vi "Agilent34410A Set AutoRange.vi"(8 "error in (no error)":errorcluster, 9 "AutoRange":bool, 10 "DMM Function":T1, 11 "VISA Rsrc":refnum<visa-resource-name>="SR530") -> (0 "error out":errorcluster, 3 "VISA Rsrc Out":refnum<visa-resource-name>="GPIB0::12::INSTR", 4 "ChaineCom":string caption="Chaîne de commande")   [LabVIEW 2019]
uses:
  <userlib>/Agilent34410A/Agilent34410A DMM_Func.ctl
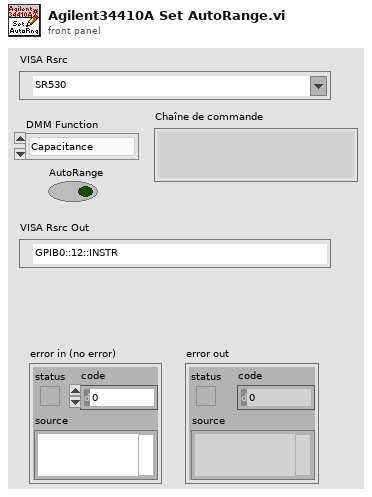
[diagram p1: front panel]
types:
  T1 = typedef "Agilent34410A DMM_Func.ctl" = enum16{"Capacitance", "Continuity", "Current AC", "Current", "Diode", "Frequency", "4W Resistance", "Period", "Resistance", "Temperature", "Voltage AC", "Voltage"}
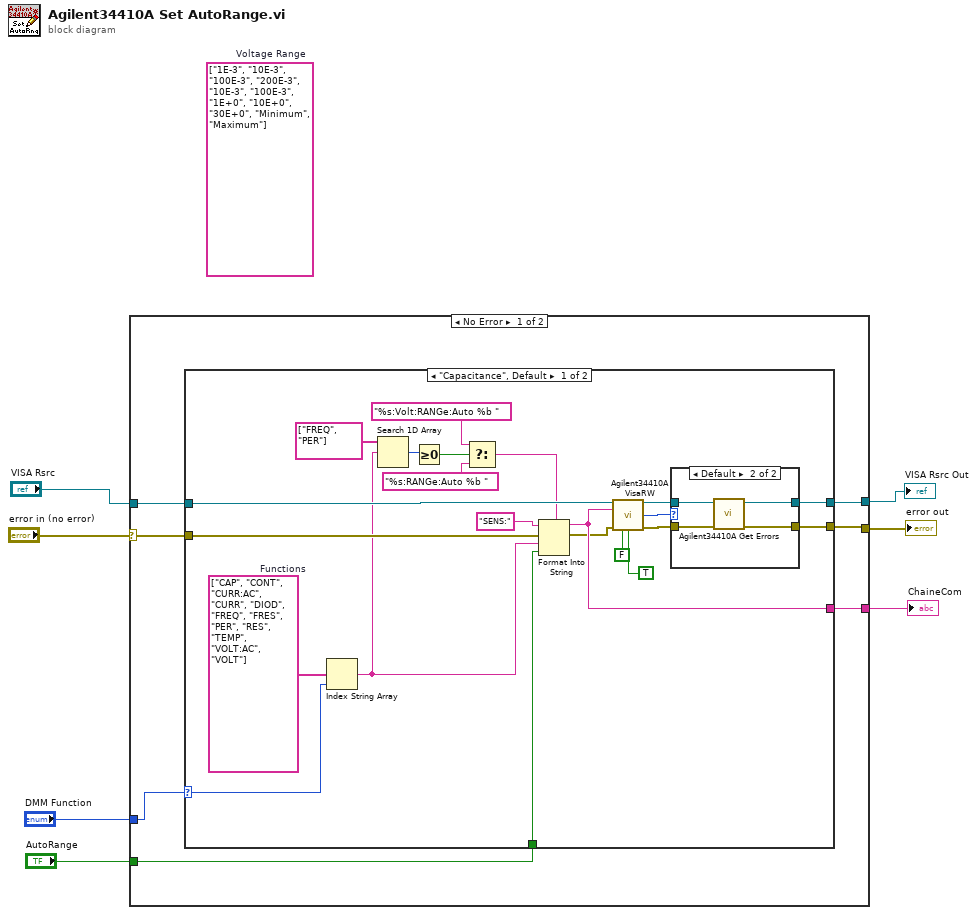
[diagram p0: block diagram]
diagram:
  (unwired) string[] ["1E-3", "10E-3", "100E-3", "200E-3", "10E-3", "100E-3", "1E+0", "10E+0", "30E+0", "Minimum", "Maximum"]  # Voltage Range
  n1 = case shown="No Error" "error in (no error)" {
    selector: "error in (no error)" -> [w12 w45]
    tunnel: "VISA Rsrc" -> [w14 w46]
    tunnel: [w11 w45] -> w5
    tunnel: [w10 w46] -> w4
    tunnel: [w13 _] -> w3
    tunnel: "DMM Function" -> [w8 _]
    tunnel: "AutoRange" -> [w9 _]
    frame No Error {
      n2 = case shown="\"Capacitance\", Default" w8 {
        selector: w8 -> [w16 _]
        tunnel: w14 -> [w36 w43]
        tunnel: [w32 _] -> w13
        tunnel: w12 -> [w31 w44]
        tunnel: [w26 w44] -> w11
        tunnel: [w25 w43] -> w10
        tunnel: w9 -> [w17 _]
        frame "Capacitance", Default {
          w35 = string[] ["CAP", "CONT", "CURR:AC", "CURR", "DIOD", "FREQ", "FRES", "PER", "RES", "TEMP", "VOLT:AC", "VOLT"]  # Functions
          n3 = Index String Array(1:w16, 2:w35) -> (0:w19:string)  [unwired: 1 in]
          n4 = Search 1D Array(1D array=string[] ["FREQ", "PER"], element=w19) -> (index of element=w23:i32)  [unwired: 1 in]
          n5 = Greater Or Equal To 0?(x=w23) -> (x >= 0?=w20:bool)
          n6 = Select(t="%s:Volt:RANGe:Auto %b " ("string (\"\")"), s=w20, f="%s:RANGe:Auto %b " ("string (\"\")")) -> (s? t:f=w18:string)
          n7 = Format Into String(format string=w18, initial string="SENS:" ("string (\"\")"), error in=w31, w19, w17) -> (resulting string=w32:string, error out=w30:errorcluster)
          n8 = call <userlib>:"Agilent34410A VisaRW.vi"("VISA Rsrc"=w36, "ChaineCom"=w32, "error in (no error)"=w30, "Lecture?(T)"=FALSE, "Poll?(F)"=TRUE) -> ("VISA Rsrc Out"=w29:refnum<visa-resource-name>, "octet d'état"=w28:u16, "error out"=w27:errorcluster)  [unwired: 6 in, 2 out]
          n9 = case shown="Default" w28 {
            tunnel: w29 -> [w38 w42]
            tunnel: w27 -> [w37 w41]
            tunnel: [w37 w40] -> w26
            tunnel: [w38 w39] -> w25
            frame 0 {
            }
            frame Default {
              n10 = call <userlib>:"Agilent34410A Get Errors.vi"("error in (no error)"=w41, "VISA Rsrc"=w42) -> ("error out"=w40:errorcluster, "VISA Rsrc Out"=w39:refnum<visa-resource-name>)  [unwired: 7 in, 1 out]
            }
          }
        }
        frame "Continuity", "Diode", "Temperature" {
        }
      }
    }
    frame Error {
    }
  }
  "error out" <- w5
  "VISA Rsrc Out" <- w4
  "ChaineCom" <- w3
